vi "BDSCTRL_Little_Endian_Bytes.vi"(8 "error in":errorcluster, 9 "Two's Complement":bool, 10 "Number of Bytes":u8=1 min=1 max=4 step=1, 11 "Value":u64) -> (0 "error out":errorcluster, 3 "Hex array":u8[](array[numeric]) format="%x")   [LabVIEW 2016]
panel:
  out "Dec array":u8[](array[numeric])
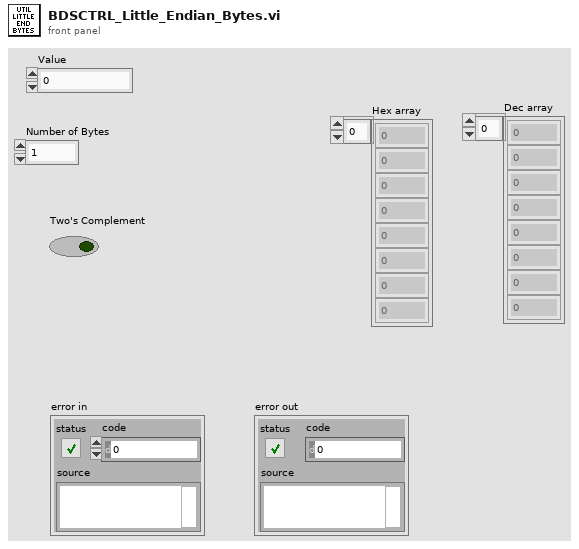
[diagram p1: front panel]
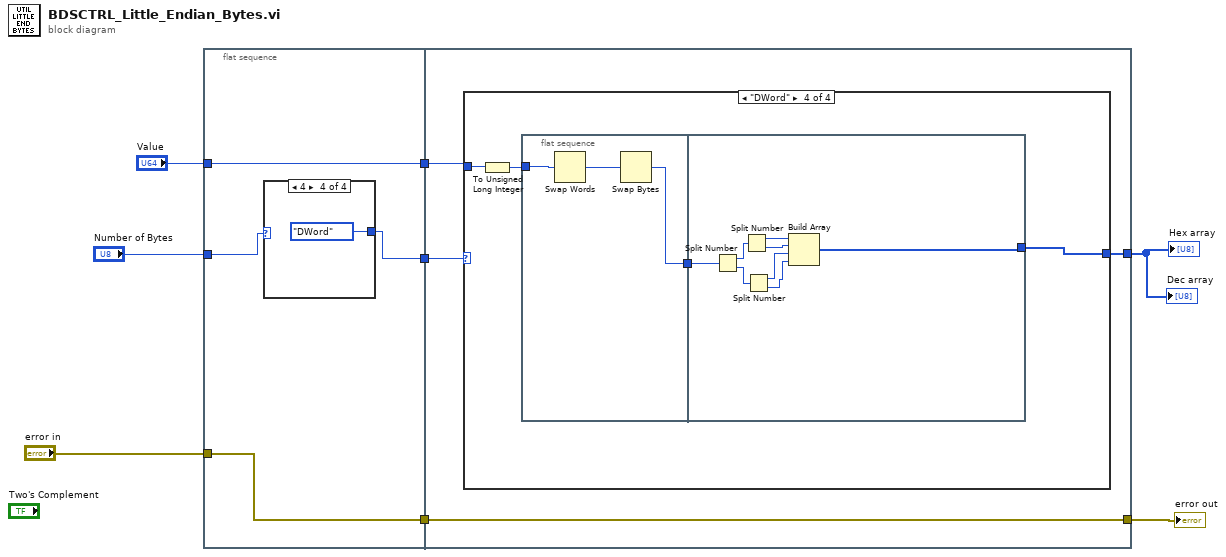
[diagram p0: block diagram]
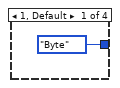
[diagram p2: hidden frame]
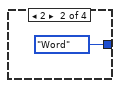
[diagram p3: hidden frame]
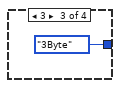
[diagram p4: hidden frame]
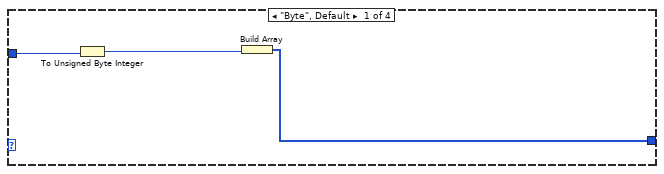
[diagram p5: hidden frame]
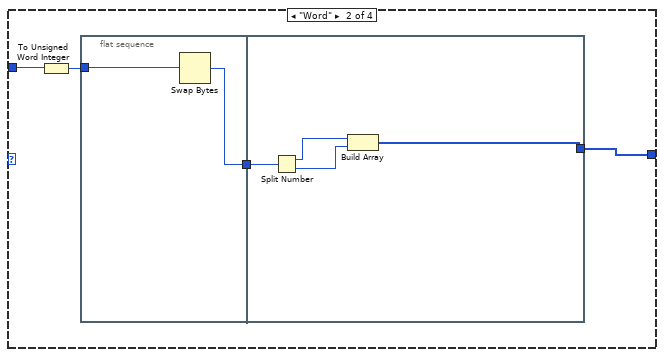
[diagram p6: hidden frame]
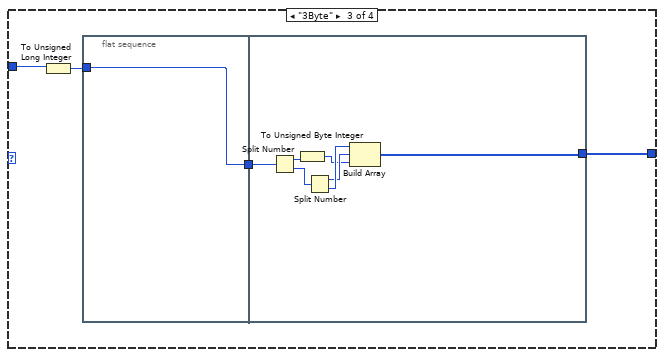
[diagram p7: hidden frame]
diagram:
  n1 = flat-sequence {
    tunnel: "Value" -> [w12]
    tunnel: [w12] -> w6
    tunnel: "Number of Bytes" -> [w11]
    tunnel: [w10] -> w4
    tunnel: "error in" -> [w9]
    tunnel: [w9] -> w2
    tunnel: [w20] -> w8
    tunnel: w6 -> [w19]
    tunnel: w4 -> [w18]
    tunnel: [w17] -> w1
    tunnel: w2 -> [w17]
    frame #0 {
      n2 = case shown="4" w11 {
        tunnel: [enum16{"Byte", "Word", "3Byte", "DWord"}."Byte" ("Bytes Number") enum16{"Byte", "Word", "3Byte", "DWord"}."Word" ("Bytes Number") enum16{"Byte", "Word", "3Byte", "DWord"}."3Byte" ("Bytes Number") enum16{"Byte", "Word", "3Byte", "DWord"}."DWord" ("Bytes Number")] -> w10
        frame 1, Default {
        }
        frame 2 {
        }
        frame 3 {
        }
        frame 4 {
        }
      }
    }
    frame #1 {
      n3 = case shown="\"DWord\"" w18 {
        tunnel: w19 -> [w22 w24 w35 w48]
        tunnel: [w23 w25 w34 w46] -> w20
        frame "Byte", Default {
          n4 = To Unsigned Byte Integer(number=w22) -> (unsigned 8bit integer=w21:u8)
          n5 = Build Array(w21) -> (w23:u8[])
        }
        frame "Word" {
          n6 = To Unsigned Word Integer(number=w24) -> (unsigned 16bit integer=w26:u16)
          n7 = flat-sequence {
            tunnel: w26 -> [w28]
            tunnel: [w29] -> w27
            tunnel: w27 -> [w33]
            tunnel: [w32] -> w25
            frame #0 {
              n8 = Swap Bytes(anything=w28) -> (byte swapped=w29:u16)
            }
            frame #1 {
              n9 = Split Number(x=w33) -> (hi(x)=w30:u8, lo(x)=w31:u8)
              n10 = Build Array(w30, w31) -> (w32:u8[])
            }
          }
        }
        frame "3Byte" {
          n11 = To Unsigned Long Integer(number=w35) -> (unsigned 32bit integer=w36:u32)
          n12 = flat-sequence {
            tunnel: w36 -> [w38]
            tunnel: [w38] -> w37
            tunnel: w37 -> [w45]
            tunnel: [w43] -> w34
            frame #0 {
            }
            frame #1 {
              n13 = Split Number(x=w45) -> (hi(x)=w40:u16, lo(x)=w44:u16)
              n14 = To Unsigned Byte Integer(number=w40) -> (unsigned 8bit integer=w39:u8)
              n15 = Split Number(x=w44) -> (hi(x)=w41:u8, lo(x)=w42:u8)
              n16 = Build Array(w42, w41, w39) -> (w43:u8[])
            }
          }
        }
        frame "DWord" {
          n17 = To Unsigned Long Integer(number=w48) -> (unsigned 32bit integer=w47:u32)
          n18 = flat-sequence {
            tunnel: w47 -> [w52]
            tunnel: [w50] -> w49
            tunnel: w49 -> [w60]
            tunnel: [w53] -> w46
            frame #0 {
              n19 = Swap Words(1:w52) -> (0:w51:u32)
              n20 = Swap Bytes(anything=w51) -> (byte swapped=w50:u32)
            }
            frame #1 {
              n21 = Split Number(x=w60) -> (hi(x)=w59:u16, lo(x)=w58:u16)
              n22 = Split Number(x=w59) -> (hi(x)=w57:u8, lo(x)=w56:u8)
              n23 = Split Number(x=w58) -> (hi(x)=w55:u8, lo(x)=w54:u8)
              n24 = Build Array(w57, w56, w55, w54) -> (w53:u8[])
            }
          }
        }
      }
    }
  }
  "Dec array" <- w8
  "Hex array" <- w8
  "error out" <- w1
